vi "Stepper FPGA 2.0.vi"() -> ()   [LabVIEW 2017]
uses:
  <vilib>/rvi/Emulation/niFpgaGetClockAttributes.vi
  <vilib>/rvi/Emulation/niFpgaSctlEmulationGetInTimedLoop.vi
  <vilib>/rvi/Emulation/niFpgaEmulationReportErrorSimple.vi
  <vilib>/rvi/eio/common/nirviEmuTemplateMethod_errors.vi
  <vilib>/rvi/Emulation/niFpgaCriticalErrorInLSC.vi
  <vilib>/eio/EIONode/EIONode.xnode
panel:
  in  "Boolean":bool
  out "Right":i64
  out "Left":i64
  in  "Right":i16
  in  "Left":i16
  in  "Motors":bool
  in  "cup size":i16
  in  "Coffee":bool
  in  "Pump":bool
  in  "Skipper":cluster{i16, i16, i16, i16, i16, i16, i16, i16}
  in  "Steps":cluster{i16, i16, i16, i16, i16, i16, i16, i16}
  out "Cluster":cluster{i16, i16, i16, i16, i16, i16, i16, i16}
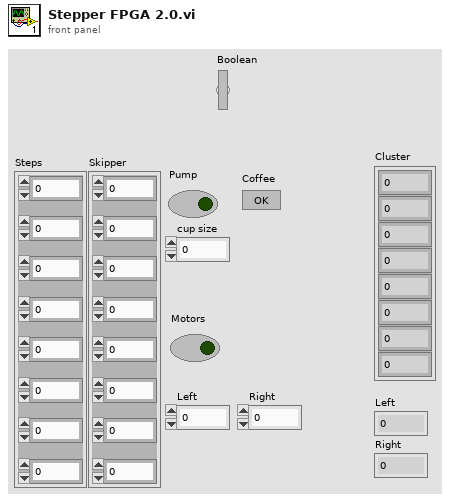
[diagram p1: front panel]
types:
  T1 = cluster{bool, bool, bool, bool, bool, bool, bool, bool}
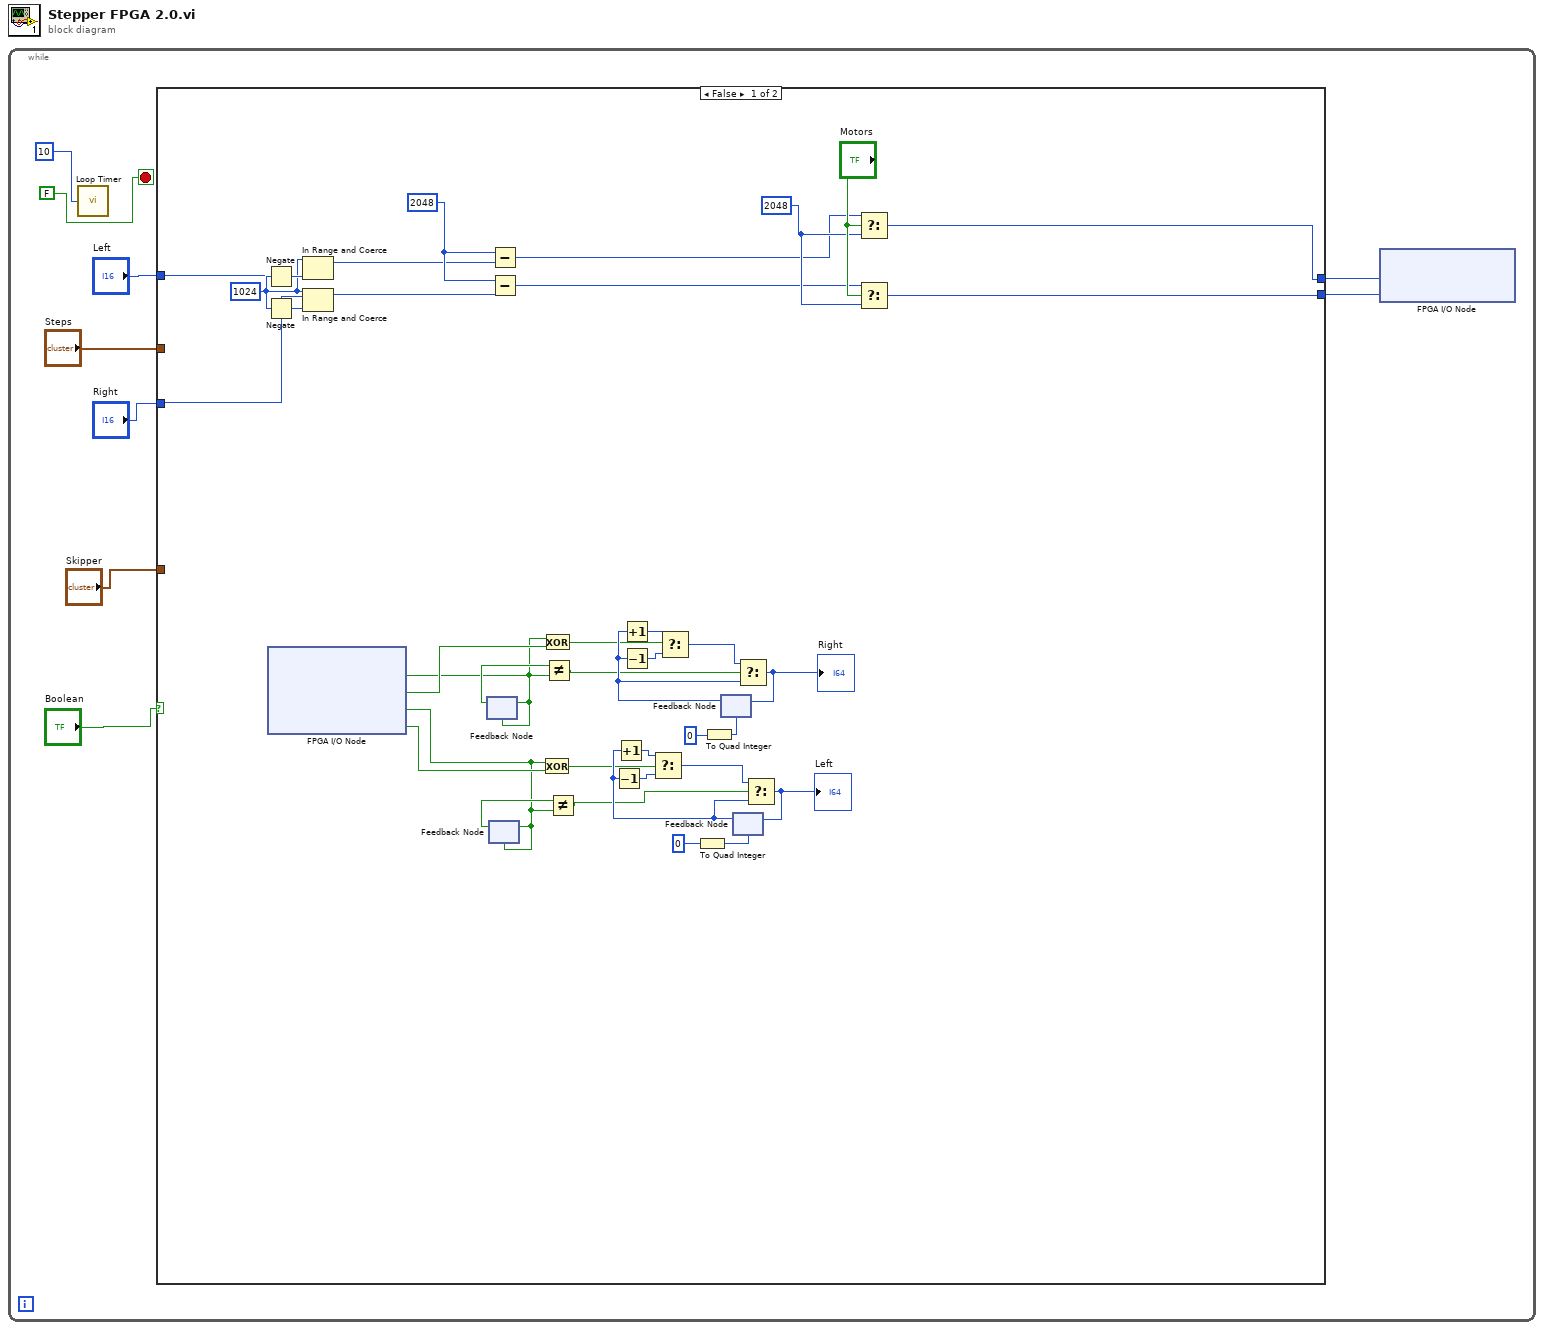
[diagram p0: block diagram]
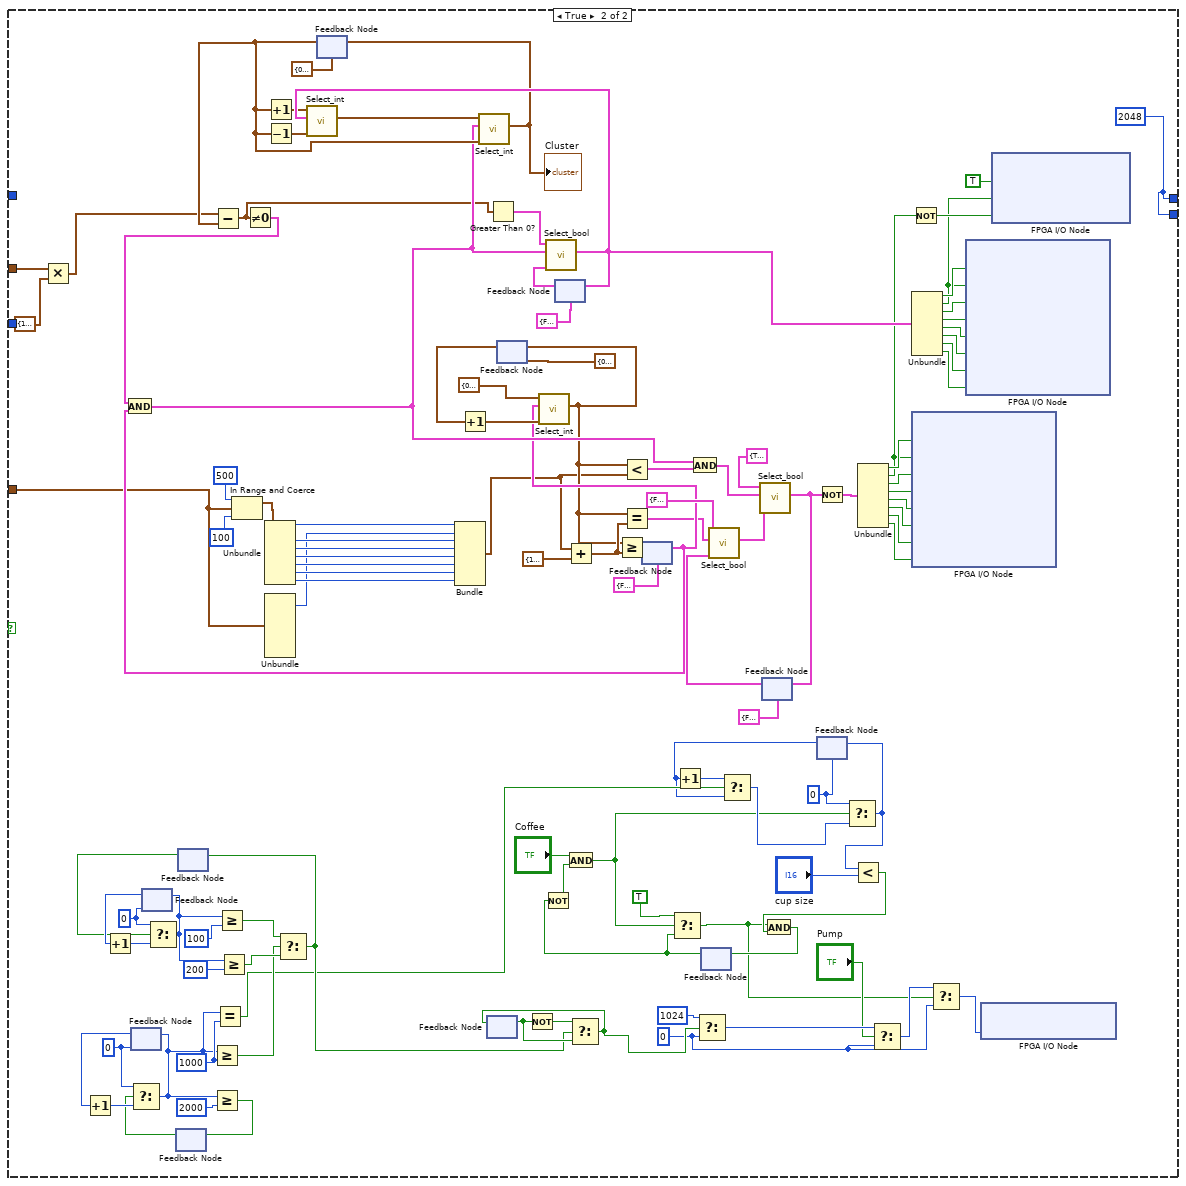
[diagram p2: hidden frame]
diagram:
  n1 = while {
    stop <- FALSE stop-if-true
    n2 = call "Loop Timer"("Count(uSec)"=u32 10) -> ()  [unwired: 1 out]
    n3 = case shown="False" "Boolean" {
      tunnel: "Steps" -> [_ w105]
      tunnel: "Skipper" -> [_ w103]
      tunnel: "Left" -> [w16 _]
      tunnel: "Right" -> [w17 _]
      tunnel: [w13 w48] -> w2
      tunnel: [w12 w48] -> w1
      frame False {
        w18 = i16 1024 ("t")
        w21 = i16 2048 ("t")
        w24 = i16 2048 ("t")
        n4 = Negate(x=w18) -> (-x=w20:i16)
        n5 = Negate(x=w18) -> (-x=w19:i16)
        n6 = xnode "FPGA I/O Node"() -> ("ConnectorC/DIO3"=w29:bool, "ConnectorC/DIO4"=w39:bool, "ConnectorC/DIO5"=w30:bool, "ConnectorC/DIO6"=w44:bool)  [unwired: 4 in, 4 out]
        n7 = In Range and Coerce(upper limit=w18, x=w16, lower limit=w20) -> (coerced(x)=w15:i16)  [unwired: 1 out]
        n8 = In Range and Coerce(upper limit=w18, x=w17, lower limit=w19) -> (coerced(x)=w14:i16)  [unwired: 1 out]
        n9 = feedback #1(w29) -> (w35:bool)
        n10 = feedback-in #1(w29) -> ()
        n11 = feedback #2(w30) -> (w40:bool)
        n12 = feedback-in #2(w30) -> ()
        n13 = Subtract(x=w21, y=w15) -> (x-y=w23:i16)
        n14 = Subtract(x=w21, y=w14) -> (x-y=w22:i16)
        n15 = Exclusive Or(1:w44, 2:w30) -> (0:w27:bool)
        n16 = Exclusive Or(1:w39, 2:w29) -> (0:w28:bool)
        n17 = Not Equal?(x=w35, y=w29) -> (x != y?=w26:bool)
        n18 = Not Equal?(x=w40, y=w30) -> (x != y?=w25:bool)
        n19 = To Quad Integer(1:i16 0) -> (0:w46:i64)
        n20 = To Quad Integer(1:i16 0) -> (0:w45:i64)
        n21 = feedback #3(w45) -> (w32:i64)
        n22 = Increment(x=w32) -> (x+1=w37:i64)
        n23 = Decrement(x=w32) -> (x-1=w36:i64)
        n24 = Select(t=w37, s=w28, f=w36) -> (s? t:f=w38:i64)
        n25 = feedback #4(w46) -> (w42:i64)
        n26 = Decrement(x=w42) -> (x-1=w31:i64)
        n27 = Increment(x=w42) -> (x+1=w41:i64)
        n28 = Select(t=w41, s=w27, f=w31) -> (s? t:f=w43:i64)
        n29 = Select(t=w38, s=w26, f=w32) -> (s? t:f=w10:i64)
        "Right" <- w10
        n30 = feedback-in #3(w10) -> ()
        n31 = Select(t=w43, s=w25, f=w42) -> (s? t:f=w11:i64)
        "Left" <- w11
        n32 = feedback-in #4(w11) -> ()
        n33 = Select(t=w23, s="Motors", f=w24) -> (s? t:f=w13:i16)
        n34 = Select(t=w22, s="Motors", f=w24) -> (s? t:f=w12:i16)
      }
      frame True {
        w48 = i16 2048 ("t")
        w68 = i16 0
        w59 = i16 1000 ("y")
        w49 = i16 0
        w83 = i16 0
        w89 = i16 0
        n35 = Multiply(x=w105, y=cluster{i16, i16, i16, i16, i16, i16, i16, i16} {1, 1, 1, 1, 1, 1, 1, 1}) -> (x*y=w106:cluster{i16, i16, i16, i16, i16, i16, i16, i16})
        n36 = feedback #5(w83) -> (w84:i16)
        n37 = Increment(x=w84) -> (x+1=w85:i16)
        n38 = feedback #6(w89) -> (w90:i16)
        n39 = Increment(x=w90) -> (x+1=w91:i16)
        n40 = feedback #7() -> (w80:bool)  [unwired: 1 in]
        n41 = Select(t=w83, s=w80, f=w85) -> (s? t:f=w58:i16)
        n42 = feedback-in #5(w58) -> ()
        n43 = feedback #8() -> (w77:bool)  [unwired: 1 in]
        n44 = Select(t=w89, s=w77, f=w91) -> (s? t:f=w88:i16)
        n45 = feedback-in #6(w88) -> ()
        n46 = Greater Or Equal?(x=w58, y=w59) -> (x >= y?=w71:bool)
        n47 = Greater Or Equal?(x=w58, y=i16 2000) -> (x >= y?=w81:bool)
        n48 = feedback-in #7(w81) -> ()
        n49 = Equal?(x=w58, y=w59) -> (x = y?=w56:bool)
        n50 = Greater Or Equal?(x=w88, y=i16 100) -> (x >= y?=w79:bool)
        n51 = Greater Or Equal?(x=w88, y=i16 200) -> (x >= y?=w78:bool)
        n52 = In Range and Coerce(upper limit=i16 500, x=w103, lower limit=i16 100) -> (coerced(x)=w102:cluster{i16, i16, i16, i16, i16, i16, i16, i16})  [unwired: 1 out]
        n53 = Unbundle(w102) -> (w101:i16, w100:i16, w99:i16, w98:i16, w97:i16, w96:i16, w95:i16)  [unwired: 1 out]
        n54 = Unbundle(w103) -> (w94:i16)  [unwired: 7 out]
        n55 = Select(t=w79, s=w71, f=w78) -> (s? t:f=w72:bool)
        n56 = feedback-in #8(w72) -> ()
        n57 = feedback #9(cluster{i16, i16, i16, i16, i16, i16, i16, i16} {0, 0, 0, 0, 0, 0, 0, 0} ("output")) -> (w152:cluster{i16, i16, i16, i16, i16, i16, i16, i16})
        n58 = Subtract(x=w106, y=w152) -> (x-y=w92:cluster{i16, i16, i16, i16, i16, i16, i16, i16})
        n59 = Not Equal To 0?(x=w92) -> (x != 0?=w118:T1)
        n60 = Increment(x=w152) -> (x+1=w155:cluster{i16, i16, i16, i16, i16, i16, i16, i16})
        n61 = Decrement(x=w152) -> (x-1=w156:cluster{i16, i16, i16, i16, i16, i16, i16, i16})
        n62 = Bundle(w101, w94, w100, w99, w98, w97, w96, w95) -> (w93:cluster{i16, i16, i16, i16, i16, i16, i16, i16})  [unwired: 1 in]
        n63 = feedback #10() -> (w74:bool)  [unwired: 1 in]
        n64 = Greater Than 0?(x=w92) -> (x > 0?=w117:T1)
        n65 = feedback #11(cluster{i16, i16, i16, i16, i16, i16, i16, i16} {0, 0, 0, 0, 0, 0, 0, 0} ("output")) -> (w147:cluster{i16, i16, i16, i16, i16, i16, i16, i16})
        n66 = Increment(x=w147) -> (x+1=w148:cluster{i16, i16, i16, i16, i16, i16, i16, i16})
        n67 = Not(x=w74) -> (.not. x?=w75:bool)
        n68 = feedback #12(T1 {FALSE, FALSE, FALSE, FALSE, FALSE, FALSE, FALSE, FALSE} ("output cluster")) -> (w151:T1)
        n69 = Add(x=w93, y=cluster{i16, i16, i16, i16, i16, i16, i16, i16} {100, 10, 100, 100, 100, 100, 100, 100}) -> (x+y=w112:cluster{i16, i16, i16, i16, i16, i16, i16, i16})
        n70 = Select(t=w75, s=w72, f=w74) -> (s? t:f=w73:bool)
        n71 = feedback-in #10(w73) -> ()
        n72 = feedback #13(T1 {FALSE, FALSE, FALSE, FALSE, FALSE, FALSE, FALSE, FALSE}) -> (w114:T1)
        n73 = And(x=w118, y=w114) -> (x .and. y?=w139:T1)
        n74 = call "Select_int.vi"("False"=w148, "Input"=w114, "True"=cluster{i16, i16, i16, i16, i16, i16, i16, i16} {0, 0, 0, 0, 0, 0, 0, 0}) -> ("output"=w111:cluster{i16, i16, i16, i16, i16, i16, i16, i16})  [unwired: 8 in]
        n75 = feedback-in #11(w111) -> ()
        n76 = call "Select_bool.vi"("False"=w151, "Input"=w139, "True"=w117) -> ("output cluster"=w158:T1)  [unwired: 8 in]
        n77 = call "Select_int.vi"("False"=w156, "Input"=w158, "True"=w155) -> ("output"=w154:cluster{i16, i16, i16, i16, i16, i16, i16, i16})  [unwired: 8 in]
        n78 = call "Select_int.vi"("False"=w152, "Input"=w139, "True"=w154) -> ("output"=w153:cluster{i16, i16, i16, i16, i16, i16, i16, i16})  [unwired: 8 in]
        "Cluster" <- w153
        n79 = feedback-in #9(w153) -> ()
        n80 = feedback-in #12(w158) -> ()
        n81 = Greater Or Equal?(x=w111, y=w112) -> (x >= y?=w116:T1)
        n82 = Less?(x=w111, y=w93) -> (x < y?=w144:T1)
        n83 = Equal?(x=w111, y=w112) -> (x = y?=w110:T1)
        n84 = feedback-in #13(w116) -> ()
        n85 = And(x=w139, y=w144) -> (x .and. y?=w143:T1)
        n86 = Select(t=i16 1024, s=w73, f=w49) -> (s? t:f=w70:i16)
        n87 = feedback #14() -> (w50:bool)  [unwired: 1 in]
        n88 = Not(x=w50) -> (.not. x?=w51:bool)
        n89 = And(x="Coffee", y=w51) -> (x .and. y?=w52:bool)
        n90 = Select(t=TRUE, s=w52, f=w50) -> (s? t:f=w60:bool)
        n91 = feedback #15(T1 {FALSE, FALSE, FALSE, FALSE, FALSE, FALSE, FALSE, FALSE} ("output cluster")) -> (w140:T1)
        n92 = call "Select_bool.vi"("False"=w140, "Input"=w110, "True"=T1 {FALSE, FALSE, FALSE, FALSE, FALSE, FALSE, FALSE, FALSE}) -> ("output cluster"=w141:T1)  [unwired: 8 in]
        n93 = call "Select_bool.vi"("False"=w141, "Input"=w143, "True"=T1 {TRUE, TRUE, TRUE, TRUE, TRUE, TRUE, TRUE, TRUE}) -> ("output cluster"=w157:T1)  [unwired: 8 in]
        n94 = feedback-in #15(w157) -> ()
        n95 = Not(x=w157) -> (.not. x?=w123:T1)
        n96 = feedback #16(w68) -> (w54:i16)
        n97 = Increment(x=w54) -> (x+1=w55:i16)
        n98 = Select(t=w55, s=w56, f=w54) -> (s? t:f=w57:i16)
        n99 = Select(t=w68, s=w52, f=w57) -> (s? t:f=w67:i16)
        n100 = feedback-in #16(w67) -> ()
        n101 = Less?(x=w67, y="cup size") -> (x < y?=w61:bool)
        n102 = And(x=w60, y=w61) -> (x .and. y?=w62:bool)
        n103 = feedback-in #14(w62) -> ()
        n104 = Unbundle(w123) -> (w124:bool, w120:bool, w130:bool, w129:bool, w128:bool, w127:bool, w126:bool, w125:bool)
        n105 = Select(t=w70, s="Pump", f=w49) -> (s? t:f=w64:i16)
        n106 = Not(x=w120) -> (.not. x?=w121:bool)
        n107 = Unbundle(w158) -> (w137:bool, w119:bool, w131:bool, w132:bool, w133:bool, w134:bool, w135:bool, w136:bool)
        n108 = xnode "FPGA I/O Node"("ConnectorA/DIO0"=w124, "ConnectorA/DIO2"=w120, "ConnectorA/DIO11"=w130, "ConnectorA/DIO5"=w129, "ConnectorA/DIO6"=w128, "ConnectorA/DIO13"=w127, "ConnectorA/DIO9"=w126, "ConnectorA/DIO14"=w125) -> ()  [unwired: 8 in, 8 out]
        n109 = Select(t=w64, s=w60, f=w49) -> (s? t:f=w65:i16)
        n110 = xnode "FPGA I/O Node"("ConnectorA/DIO1"=w137, "ConnectorA/DIO3"=w119, "ConnectorA/DIO4"=w131, "ConnectorA/DIO12"=w132, "ConnectorA/DIO7"=w133, "ConnectorA/DIO8"=w134, "ConnectorA/DIO10"=w135, "ConnectorA/DIO15"=w136) -> ()  [unwired: 8 in, 8 out]
        n111 = xnode "FPGA I/O Node"("ConnectorC/AO1"=w65) -> ()  [unwired: 1 in, 1 out]
        n112 = xnode "FPGA I/O Node"("ConnectorC/DIO0"=TRUE, "ConnectorC/DIO1"=w119, "ConnectorC/DIO2"=w121) -> ()  [unwired: 3 in, 3 out]
      }
    }
    n113 = xnode "FPGA I/O Node"("ConnectorA/AO0"=w2, "ConnectorA/AO1"=w1) -> ()  [unwired: 2 in, 2 out]
  }
